vi "Calibration Filename (Set).vi"(6 "ISOBUS address":T3=-1 caption="ISOBUS address (-1)", 8 "error in":errorcluster, 10 "Filename":string, 11 "Mercury Reference In":T4) -> (0 "error out":errorcluster, 2 "Response":T1, 3 "Mercury Reference Out":T4, 4 "Valid?":T2)   [LabVIEW 2015, in "Mercury iXX.lvlib" / "Pressure.lvlib"]
doc: "Set the current calibration file for the selected pressure device."
uses:
  Pressure.lvlib
  Controls/Mercury Reference.ctl
  Controls/Comms Transport Layer.ctl
  Private/Controls/Query Dynamic Reference.ctl
  Controls/ISOBus Address.ctl
  Controls/Is Valid LED.ctl
  Controls/Response String.ctl
  Private/Controls/Command Verbs.ctl
  Mercury iXX.lvlib
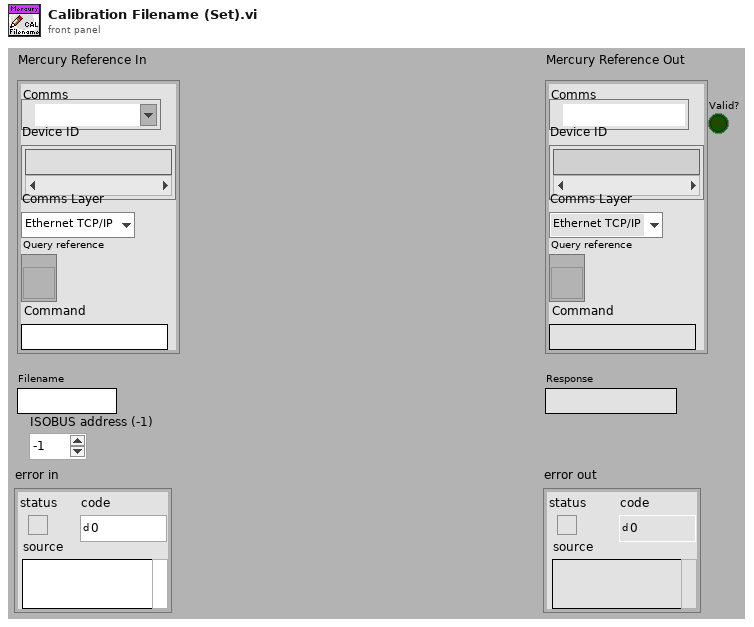
[diagram p1: front panel]
types:
  T1 = typedef "Mercury iXX.lvlib/Response String.ctl" = string
  T2 = typedef "Mercury iXX.lvlib/Is Valid LED.ctl" = bool
  T3 = typedef "Mercury iXX.lvlib/ISOBus Address.ctl" = i32
  T4 = typedef "Mercury iXX.lvlib/Mercury Reference.ctl" = cluster{"Comms":refnum<visa-resource-name>, "Device ID":string[], "Comms Layer":T5, "Command":string, "Query reference":T6}
  T5 = typedef "Mercury iXX.lvlib/Comms Transport Layer.ctl" = enum16{"Ethernet TCP/IP", "USB", "ISOBus - RS-232", "GPIB"}
  T6 = typedef "Mercury iXX.lvlib/Query Dynamic Reference.ctl" = refnum<vi>
  T7 = typedef "Mercury iXX.lvlib/Command Verbs.ctl" = string
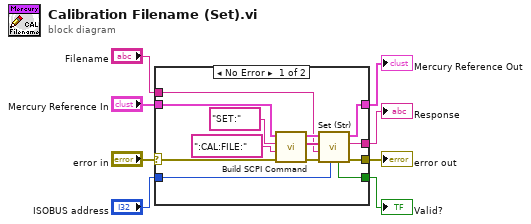
[diagram p0: block diagram]
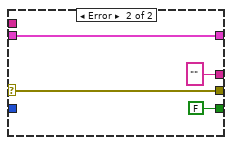
[diagram p2: hidden frame]
diagram:
  n1 = case shown="No Error" "error in" {
    selector: "error in" -> [w9 w24]
    tunnel: [w11 T1 "" ("Response")] -> w8
    tunnel: "Filename" -> [w10 _]
    tunnel: "Mercury Reference In" -> [w16 w25]
    tunnel: [w15 w25] -> w5
    tunnel: [w14 w24] -> w4
    tunnel: [w13 T2 FALSE ("Valid?")] -> w3
    tunnel: "ISOBUS address" -> [w12 _]
    frame No Error {
      n2 = call "Build SCPI Command.vi"("error in"=w9, "Noun(s)"=":CAL:FILE:" ("Command"), "Verb"=T7 "SET:", "Mercury Reference In"=w16) -> ("error out"=w18:errorcluster, "SCPI Message(s)"=w19:string[], "Mercury Reference Out"=w20:T4)  [unwired: 5 out]
      n3 = call "Set (Str).vi"("ISOBUS address"=w12, "error in"=w18, "Command Value (Str)"=w10, "SCPI Message(s)"=w19, "Mercury Reference In"=w20) -> ("error out"=w14:errorcluster, "Response"=w11:T1, "Mercury Reference Out"=w15:T4, "Valid?"=w13:T2)  [unwired: 3 out]
    }
    frame Error {
    }
  }
  "Mercury Reference Out" <- w5
  "error out" <- w4
  "Valid?" <- w3
  "Response" <- w8
